vi "Make_Dots_Status_Zero_after_Removal-1.vi"(1 "# Frame":i32, 2 "# Dot":i32, 3 "[IN] Dot matrix\nwith initial status":i16[][](array[numeric])) -> (0 "[IN] Dot matrix\nwith zero deleted\ndots":i16[][](array[numeric]))   [LabVIEW 2013]
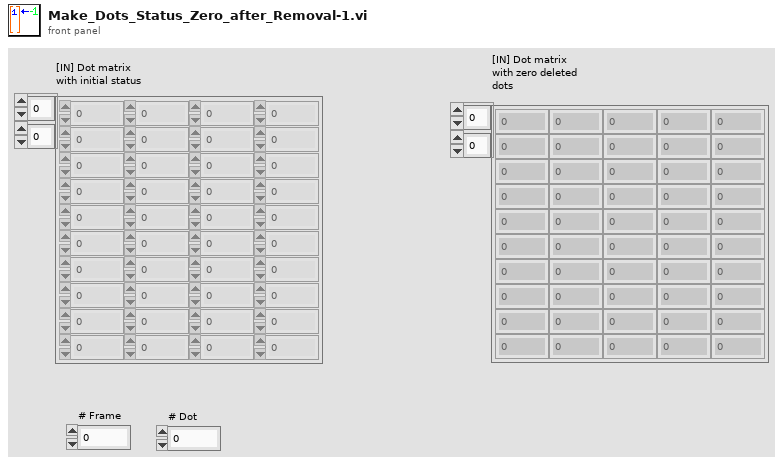
[diagram p1: front panel]
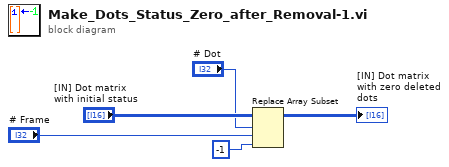
[diagram p0: block diagram]
diagram:
  n1 = Replace Array Subset(array="[IN] Dot matrix\nwith initial status", new element=i16 -1 ("new element/subarray"), index (row)="# Dot", index (col)="# Frame") -> (→"[IN] Dot matrix\nwith zero deleted\ndots":i16[][])
